vi "Position A.vi"(8 "error in (no error)":errorcluster, 11 "VICI Electronic Actuator In":T1) -> (0 "error out":errorcluster, 1 "Initialized":bool, 2 "No Pump Connected":bool, 3 "VICI Electronic Actuator Out":T1)   [LabVIEW 2021, in "VICI Electronic Actuator.lvlib"]
uses:
  D-O Module Folder/DIO Valve/VICI Electronic Actuator.lvlib
  VICI Electronic Actuator Settings.ctl
  <vilib>/Instr/_visa.llb/VISA Configure Serial Port (Instr).vi
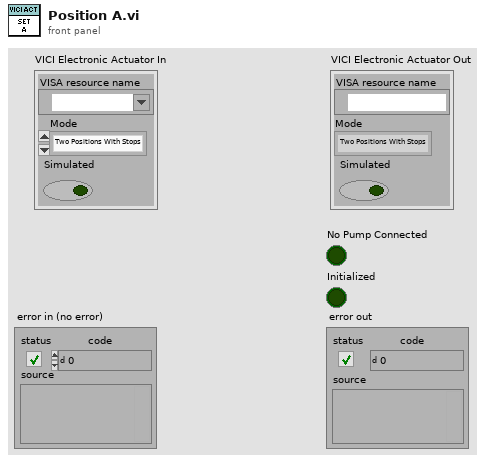
[diagram p1: front panel]
types:
  T1 = typedef "VICI Electronic Actuator.lvlib/VICI Electronic Actuator Settings.ctl" = cluster{"VISA resource name":refnum<visa-resource-name>, "Mode":enum16{"Two Positions With Stops", "Two Positions Without Stops", "Mutiposition"}, "Simulated":bool}
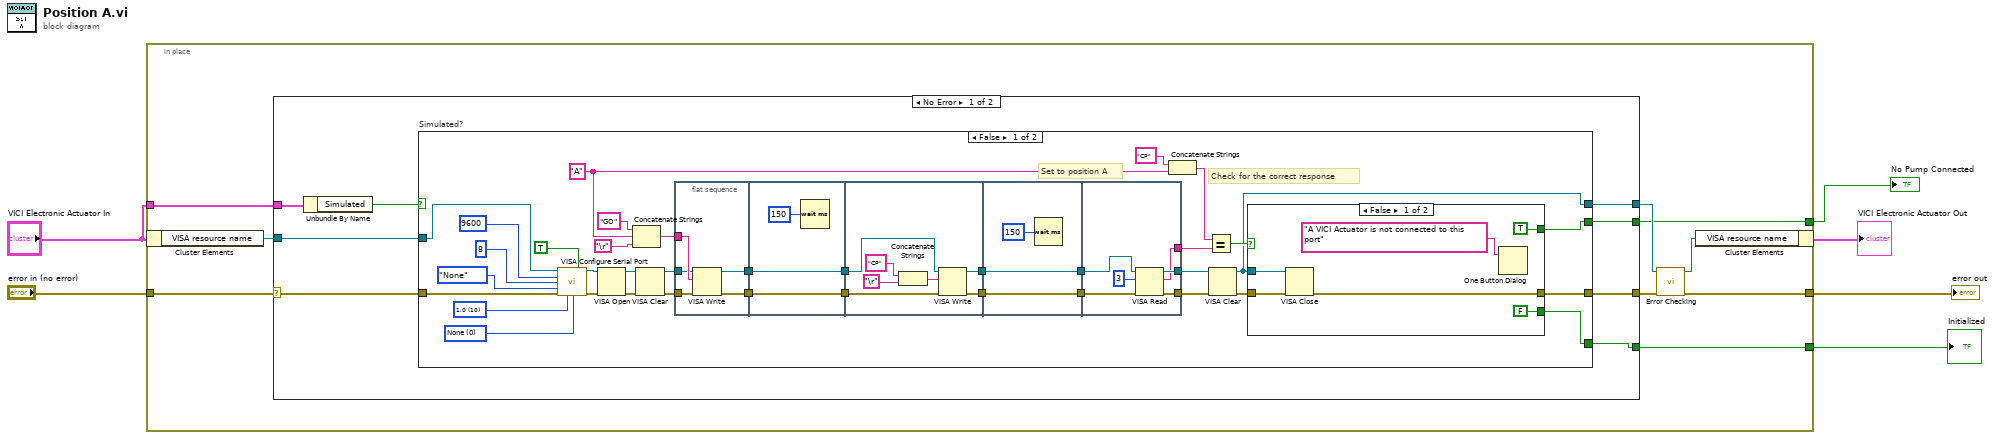
[diagram p0: block diagram]
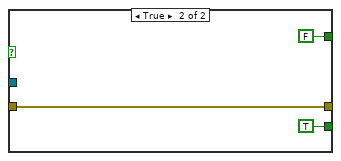
[diagram p2: hidden frame]
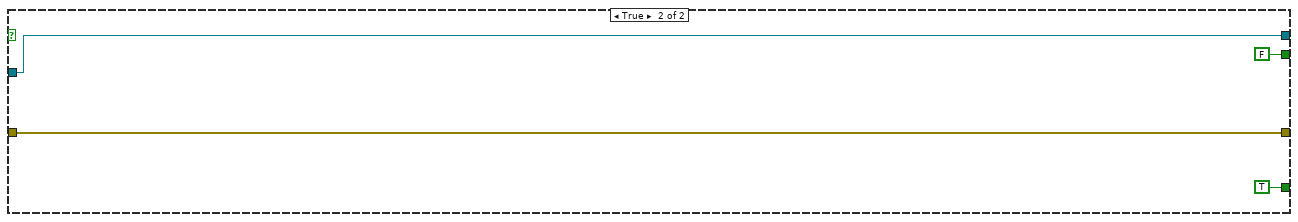
[diagram p3: hidden frame]
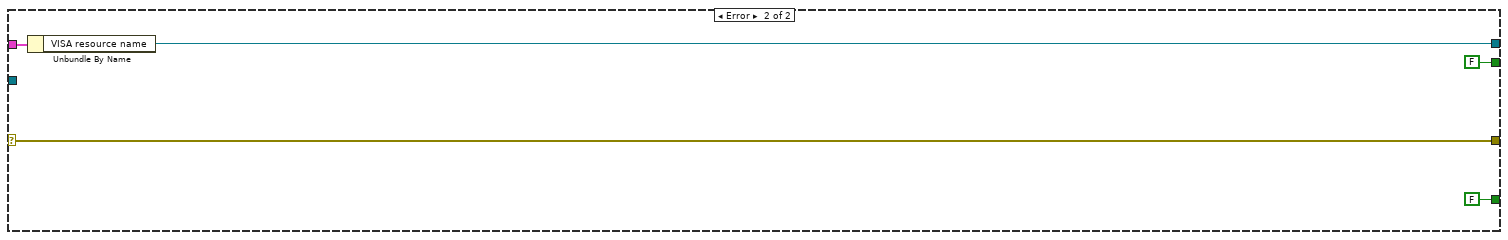
[diagram p4: hidden frame]
diagram:
  n1 = in-place {
    in-place-border: "error in (no error)" -> [w15]
    in-place-border: [w12] -> w5
    in-place-border: [w11] -> w4
    in-place-border: "VICI Electronic Actuator In" -> [w10]
    in-place-border: [w9] -> w3
    n2 = in-place-cluster #1("VICI Electronic Actuator In") -> ("VISA resource name"=w8:refnum<visa-resource-name>)
    n3 = case shown="No Error" w15 {
      selector: w15 -> [w23 w102]
      tunnel: w10 -> [w20 w101]
      tunnel: [w21 w102] -> w13
      tunnel: [w19 w100] -> w14
      tunnel: [w18 FALSE] -> w11
      tunnel: [w17 FALSE] -> w9
      tunnel: w8 -> [w16 _]
      frame No Error {
        n4 = Unbundle By Name(w20) -> ("Simulated"=w22:bool)
        n5 = case "Simulated?" shown="False" w22 {
          tunnel: w23 -> [w54 w97]
          tunnel: [w45 w97] -> w21
          tunnel: [w50 w96] -> w19
          tunnel: w16 -> [w52 w96]
          tunnel: [w44 TRUE] -> w18
          tunnel: [w24 FALSE] -> w17
          frame False {
            w31 = "A"
            w56 = u16 0 items=["None", "XON/XOFF", "RTS/CTS", "XON/XOFF & RTS/CTS", "DTR/DSR", "XON/XOFF & DTR/DSR"] ("flow control (0:none)")
            w57 = u16 10 items=["1.0"=10, "1.5"=15, "2.0"=20] ("stop bits (10: 1 bit)")
            # "Check for the correct response"
            # "Set to position A"
            n6 = call-poly "VISA Configure Serial Port"("VISA resource name"=w52, "Enable Termination\nChar (T)"=TRUE ("Enable Termination\nChar (T)"), "baud rate (9600)"=u32 9600, "data bits (8)"=u16 8, "parity (0:none)"=enum16{"None", "Odd", "Even", "Mark", "Space"}."None", "error in (no error)"=w54, "stop bits (10: 1 bit)"=w57, "flow control (0:none)"=w56) -> ("VISA resource name out"=w53:refnum<visa-resource-name>, "error out"=w55:errorcluster)  [unwired: 6 in]
            n7 = VISA Open(error in (no error)=w55, VISA resource name=w53) -> (VISA resource name=w49:refnum<visa-resource-name>, error out=w48:errorcluster)  [unwired: 3 in]
            n8 = Concatenate Strings("GO" ("string"), w31, "\r") -> (w35:string)
            n9 = VISA Clear(VISA resource name=w49, error in (no error)=w48) -> (VISA resource name out=w34:refnum<visa-resource-name>, error out=w36:errorcluster)
            n10 = flat-sequence {
              tunnel: [w61] -> w43
              tunnel: [w62] -> w42
              tunnel: w36 -> [w65]
              tunnel: w35 -> [w64]
              tunnel: w34 -> [w63]
              tunnel: [w67] -> w30
              tunnel: w43 -> [w67]
              tunnel: w42 -> [w66]
              tunnel: [w66] -> w29
              tunnel: w30 -> [w75]
              tunnel: [w73] -> w28
              tunnel: w29 -> [w74]
              tunnel: [w72] -> w26
              tunnel: w28 -> [w78]
              tunnel: [w78] -> w27
              tunnel: w26 -> [w77]
              tunnel: [w77] -> w25
              tunnel: [w84] -> w37
              tunnel: [w83] -> w38
              tunnel: w27 -> [w81]
              tunnel: w25 -> [w80]
              tunnel: [w79] -> w40
              frame #0 {
                n11 = VISA Write(VISA resource name=w63, write buffer=w64, error in (no error)=w65) -> (VISA resource name out=w61:refnum<visa-resource-name>, error out=w62:errorcluster)  [unwired: 1 out]
              }
              frame #1 {
                n12 = Wait (ms)(milliseconds to wait=u32 150) -> ()  [unwired: 1 out]
              }
              frame #2 {
                n13 = Concatenate Strings("CP" ("write buffer"), "\r") -> (w70:string)
                n14 = VISA Write(VISA resource name=w75, write buffer=w70, error in (no error)=w74) -> (VISA resource name out=w73:refnum<visa-resource-name>, error out=w72:errorcluster)  [unwired: 1 out]
              }
              frame #3 {
                n15 = Wait (ms)(milliseconds to wait=u32 150) -> ()  [unwired: 1 out]
              }
              frame #4 {
                n16 = VISA Read(VISA resource name=w81, byte count=u32 3, error in (no error)=w80) -> (VISA resource name out=w83:refnum<visa-resource-name>, read buffer=w79:string, error out=w84:errorcluster)  [unwired: 1 out]
              }
            }
            n17 = Concatenate Strings("CP" ("string"), w31) -> (w39:string)
            n18 = Equal?(x=w39, y=w40) -> (x = y?=w51:bool)
            n19 = VISA Clear(VISA resource name=w38, error in (no error)=w37) -> (VISA resource name out=w50:refnum<visa-resource-name>, error out=w46:errorcluster)
            n20 = case shown="False" w51 {
              tunnel: w50 -> [w89 _]
              tunnel: w46 -> [w88 w92]
              tunnel: [TRUE FALSE] -> w24
              tunnel: [w86 w92] -> w45
              tunnel: [FALSE TRUE] -> w44
              frame False {
                n21 = VISA Close(VISA resource name=w89, error in (no error)=w88) -> (error out=w86:errorcluster)
                n22 = One Button Dialog(message="A VICI Actuator is not connected to this port") -> ()  [unwired: 1 in, 1 out]
              }
              frame True {
              }
            }
          }
          frame True {
          }
        }
      }
      frame Error {
        n23 = Unbundle By Name(w101) -> ("VISA resource name"=w100:refnum<visa-resource-name>)
      }
    }
    n24 = call "Error Checking.vi"("error in (no error)"=w13, "VISA resource name"=w14) -> ("error out"=w12:errorcluster, "VISA resource name"=w7:refnum<visa-resource-name>)  [unwired: 7 in, 1 out]
    n25 = in-place-cluster #1("VISA resource name"=w7) -> (→"VICI Electronic Actuator Out":T1)
  }
  "error out" <- w5
  "Initialized" <- w4
  "No Pump Connected" <- w3
